vi "SwerveDrivePoseEst_New.vi"(4 "ModulePositions":T1[](array[typedef]) {"Angle"."SIN" format="%13.4f"; "Angle"."COS" format="%13.4f"; "Angle"."VALUE" format="%13.4f"}, 5 "gyroAngle":T2={"VALUE"=0.0, "COS"=1.0, "SIN"=0.0} {"SIN" format="%13.4f"; "COS" format="%13.4f"; "VALUE" format="%13.4f"}, 6 "SwerveKinematics":T3 {"SavedModuleStates"."Angle"."SIN" format="%13.4f"; "SavedModuleStates"."Angle"."COS" format="%13.4f"; "SavedModuleStates"."Angle"."VALUE" format="%13.4f"; "PrevCoR"."Y" format="%14.3f"; "PrevCoR"."X" format="%14.3f"; "Modules"."Y" format="%14.3f"; "Modules"."X" format="%14.3f"}, 7 "InitialPose":T7={"TRANSLATION"={"X"=0.0, "Y"=0.0}, "ROTATION"={"VALUE"=0.0, "COS"=1.0, "SIN"=0.0}} {"ROTATION"."SIN" format="%13.4f"; "ROTATION"."COS" format="%13.4f"; "ROTATION"."VALUE" format="%13.4f"; "TRANSLATION"."Y" format="%14.3f"; "TRANSLATION"."X" format="%14.3f"}, 8 "dt_Seconds":dbl=0.02, 9 "VisionMeasurementStdDevs":T4, 10 "LocalMeasurementStdDevs":T4, 11 "StateStdDevs":T4) -> (0 "Error":errorcluster, 3 "SwerveDrivePoseEstimate":T8={"M_VisionContR"=[], "m_nominal_dT"=0.0, "m_PrevTime_Sec"=0.0, "m_GyroOffset"={"VALUE"=0.0, "COS"=1.0, "SIN"=0.0}, "m_PrevAngle"={"VALUE"=0.0, "COS"=1.0, "SIN"=0.0}, "m_Observer"={"m_P"=[], "m_xHat"=[], "States"=0, "Outputs"=0, "m_ContR"=[], "m_ContQ"=[], "m_SigmasF"=[], "m_dT_Sec"=0.0, "MERWE_SCALED_SIGMA_PTS"={"m_Wm"=[], "States"=0, "Alpha"=0.0, "m_Wc"=[], "Kappa"=0}, "meanFuncX"=refnum, "meanFuncY"=refnum, "residualFuncX"=refnum, "residualFuncY"=refnum, "addFuncX"=refnum, "addFuncXExtra"=variant, "residualFuncYExtra"=variant, "residualFuncXExtra"=variant, "MeanFuncYExtra"=variant, "MeanFuncXExtra"=variant, "Inputs"=0}, "m_kinematics"={"NumModules"=0, "InverseKinematics"=[], "ForwardKinematics"=[], "Modules"=[], "PrevCoR"={"X"=0.0, "Y"=0.0}, "SavedModuleStates"=[]}, "Pose_Buffer"={"TimeStamps"=[], "Pose"=[], "Min_TimeStamp"=0.0, "Max_TimeStamp"=0.0, "ItemCount"=0, "MaxBufferTime"=0.0}, "States"=0, "Inputs"=0, "Outputs"=0} {"Pose_Buffer"."Pose"."ROTATION"."SIN" format="%13.4f"; "Pose_Buffer"."Pose"."ROTATION"."COS" format="%13.4f"; "Pose_Buffer"."Pose"."ROTATION"."VALUE" format="%13.4f"; "Pose_Buffer"."Pose"."TRANSLATION"."Y" format="%14.3f"; "Pose_Buffer"."Pose"."TRANSLATION"."X" format="%14.3f"; "m_kinematics"."SavedModuleStates"."Angle"."SIN" format="%13.4f"; "m_kinematics"."SavedModuleStates"."Angle"."COS" format="%13.4f"; "m_kinematics"."SavedModuleStates"."Angle"."VALUE" format="%13.4f"; "m_kinematics"."PrevCoR"."Y" format="%14.3f"; "m_kinematics"."PrevCoR"."X" format="%14.3f"; "m_kinematics"."Modules"."Y" format="%14.3f"; "m_kinematics"."Modules"."X" format="%14.3f"; "m_PrevAngle"."SIN" format="%13.4f"; "m_PrevAngle"."COS" format="%13.4f"; "m_PrevAngle"."VALUE" format="%13.4f"; "m_GyroOffset"."SIN" format="%13.4f"; "m_GyroOffset"."COS" format="%13.4f"; "m_GyroOffset"."VALUE" format="%13.4f"})   [LabVIEW 2019, in "Trajectory_Library.lvlib"]
doc: "Constructs a SwerveDrivePoseEstimator.\n\nThis class wraps an UnscentedKalmanFilter Unscented Kalman Filter to fuse latency-compensated vision measurements with swerve drive encoder velocity measurements. It will correct for noisy measurements and encoder drift. It is intended to be an easy but more accurate drop-in for SwerveDriveOdometry.\n \nSwerveDrivePoseEstimator_update should be called every robot loop. If your loops are faster or slower than the default of 0.02s, then you should change the nominal delta time using the calling parameter. \n \nSwerveDrivePoseEstimator_addVisionMeasurement can be called as infrequently as you want; if you never call it, then this class will behave mostly like regular encoder odometry.\n \nThe state-space system used internally has the following states (x), inputs (u), and outputs\n(y):\n \n x = [x, y, theta]? \n in the field coordinate system containing x position, \n y position, and heading.\n \n u = [v_l, v_r, dtheta]? \n containing left wheel velocity, right wheel velocity, \n and change in gyro heading.\n \n y = [x, y, theta]?\n from vision containing x position, y position, and\n heading; or <strong> y = [theta]? </strong> containing \n gyro heading.\n \n \nInputs:\n - gyroAngle -- The current gyro angle.\n - initialPoseMeters -- The starting pose estimate.\n - stateStdDevs -- Standard deviations of model states. Increase these numbers \n to trust your model's state estimates less. This matrix is in the form \n [x, y, theta]?, with units in meters and radians.\n - localMeasurementStdDevs -- Standard deviations of the encoder and gyro \n measurements. Increase these numbers to trust sensor readings from encoders \n and gyros less. This matrix is in the form [theta], with units in radians.\n - visionMeasurementStdDevs -- Standard deviations of the vision measurements. \n Increase these numbers to trust global measurements from vision less. \n This matrix is in the form [x, y,theta]?, with units in meters and radians.\n - nominalDtSeconds -- The time in seconds between each robot loop.\n - SwerveKinematics -- A correctly-configured kinematics object for your drivetrain.\n\n\nOutputs:\n - outSwevePoseEst -- Updated data cluster \n - Error -- If TRUE, an error occured."
uses:
  Trajectory_Library.lvlib
  TypeDef/SWERVE_DRIVE_POSE_EST.ctl
  <vilib>/Analysis/Matrix/Datatypes/RealMatrix.ctl
  TypeDef/ROTATION2D.ctl
  TypeDef/UNSCENTED_KALMAN_FILTER.ctl
  TypeDef/MERWE_SCALED_SIGMA_PTS.ctl
  TypeDef/CALLBACK_FUNC_TYPE.ctl
  TypeDef/SWERVE_DRIVE_KINEMATICS.ctl
  TypeDef/TRANSLATION2D.ctl
  TypeDef/SWERVE_DRIVE_MODULE_STATE.ctl
  TypeDef/TIME_INTERPOLATABLE_POSE2D.ctl
  TypeDef/POSE2D.ctl
  MatBuilder_Create.vi
  VecBuilder_3x1Fill.vi
  Pose2d_getXYAngle.vi
  Rotation2d_UnaryMinus.vi
  Rotation2d_RotateBy.vi
  Rotation2d_CreateAngle.vi
  Rotation2d_CreateXY.vi
  Util_CalcDist.vi
  <vilib>/Analysis/Matrix/NI_Matrix.lvlib
  TypeDef/SWERVE_DRIVE_MODULE_POSITION.ctl
panel:
  in  "RightDistance_M":dbl=0.02
  in  "LeftDistance_M":dbl=0.02
  # "<5,1>"
  # "<3, 1>"
  # "<3, 1>"
  # "<3, 3>"
  # "State Estimate <Statess,1>"
  # "<States, States>"
  # "<States, ?>"
  # "<Statess,  States>"
  # "<Outputs, Outputs>"
  # "<?, 1>"
  # "<?, 1>"
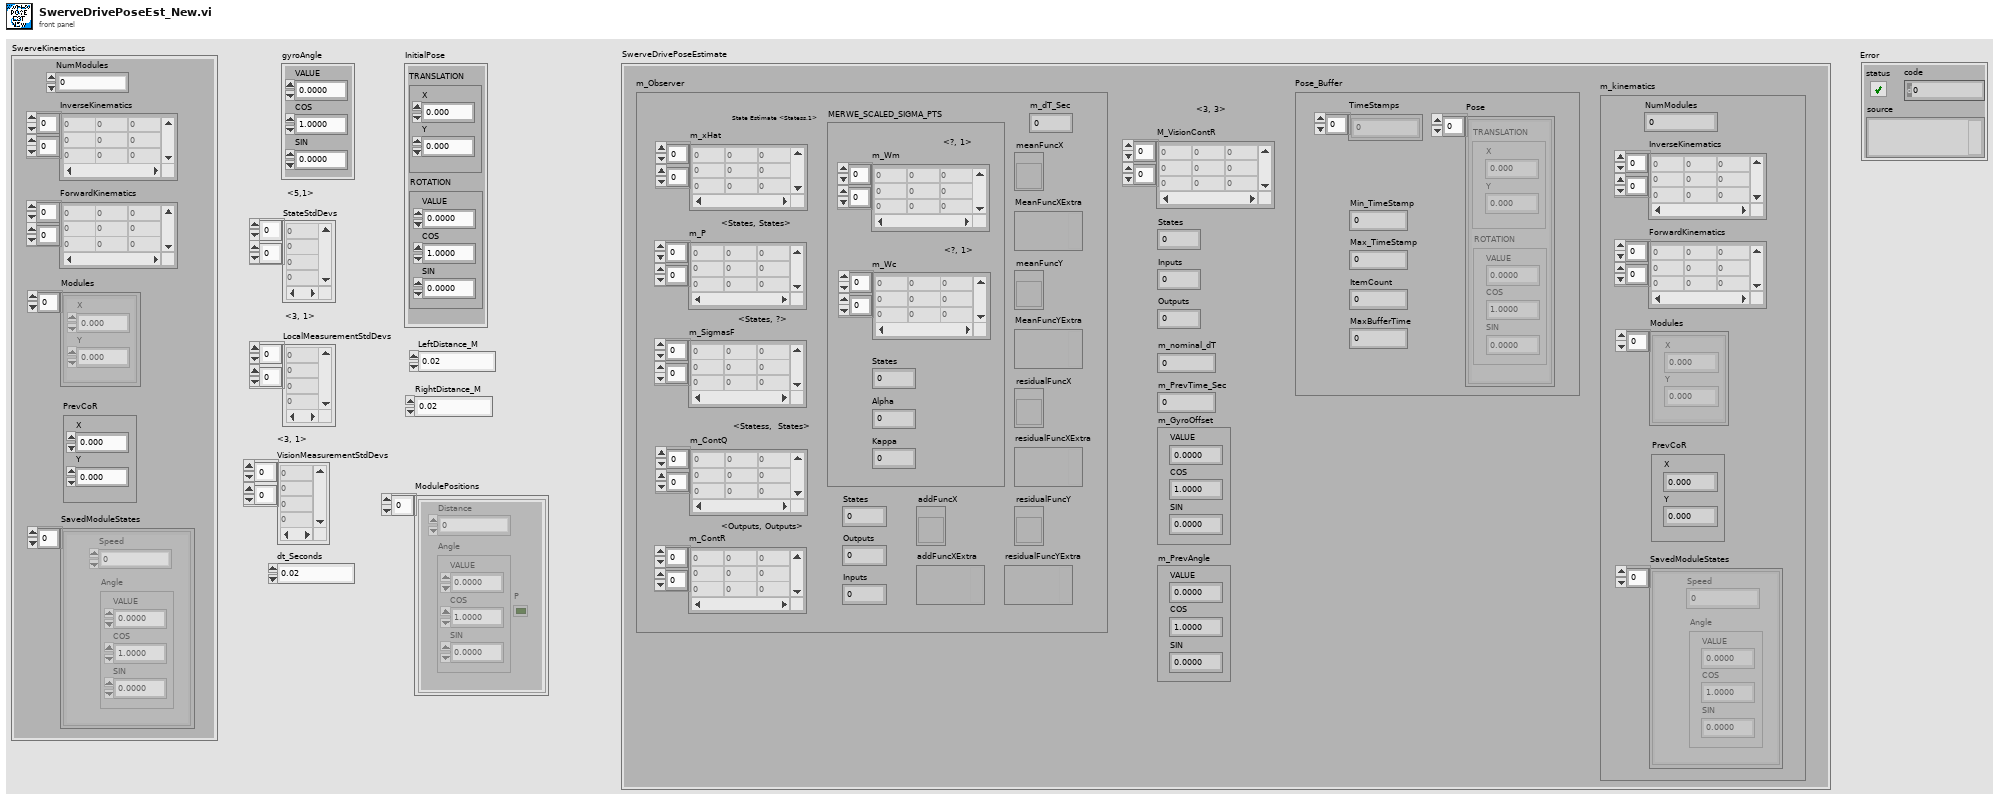
[diagram p1: front panel]
types:
  T1 = typedef "Trajectory_Library.lvlib/SWERVE_DRIVE_MODULE_POSITION.ctl" = cluster{"Distance":dbl, "Angle":T2, "P":bool}
  T2 = typedef "Trajectory_Library.lvlib/ROTATION2D.ctl" = cluster{"VALUE":dbl, "COS":dbl, "SIN":dbl}
  T3 = typedef "Trajectory_Library.lvlib/SWERVE_DRIVE_KINEMATICS.ctl" = cluster{"NumModules":i32, "InverseKinematics":T4, "ForwardKinematics":T4, "Modules":T5[], "PrevCoR":T5, "SavedModuleStates":T6[]}
  T4 = typedef "NI_Matrix.lvlib/RealMatrix.ctl" = dbl[][]
  T5 = typedef "Trajectory_Library.lvlib/TRANSLATION2D.ctl" = cluster{"X":dbl, "Y":dbl}
  T6 = typedef "Trajectory_Library.lvlib/SWERVE_DRIVE_MODULE_STATE.ctl" = cluster{"Speed":dbl, "Angle":T2}
  T7 = typedef "Trajectory_Library.lvlib/POSE2D.ctl" = cluster{"TRANSLATION":T5, "ROTATION":T2}
  T8 = typedef "Trajectory_Library.lvlib/SWERVE_DRIVE_POSE_EST.ctl" = cluster{"M_VisionContR":T4, "m_nominal_dT":dbl, "m_PrevTime_Sec":dbl, "m_GyroOffset":T2, "m_PrevAngle":T2, "m_Observer":T9, "m_kinematics":T3, "Pose_Buffer":T12, "States":i32, "Inputs":i32, "Outputs":i32}
  T9 = typedef "Trajectory_Library.lvlib/UNSCENTED_KALMAN_FILTER.ctl" = cluster{"m_P":T4, "m_xHat":T4, "States":i32, "Outputs":i32, "m_ContR":T4, "m_ContQ":T4, "m_SigmasF":T4, "m_dT_Sec":dbl, "MERWE_SCALED_SIGMA_PTS":T10, "meanFuncX":T11, "meanFuncY":T11, "residualFuncX":T11, "residualFuncY":T11, "addFuncX":T11, "addFuncXExtra":variant, "residualFuncYExtra":variant, "residualFuncXExtra":variant, "MeanFuncYExtra":variant, "MeanFuncXExtra":variant, "Inputs":i32}
  T10 = typedef "Trajectory_Library.lvlib/MERWE_SCALED_SIGMA_PTS.ctl" = cluster{"m_Wm":T4, "States":i32, "Alpha":dbl, "m_Wc":T4, "Kappa":i32}
  T11 = typedef "Trajectory_Library.lvlib/CALLBACK_FUNC_TYPE.ctl" = refnum<vi>
  T12 = typedef "Trajectory_Library.lvlib/TIME_INTERPOLATABLE_POSE2D.ctl" = cluster{"TimeStamps":dbl[], "Pose":T7[], "Min_TimeStamp":dbl, "Max_TimeStamp":dbl, "ItemCount":i32, "MaxBufferTime":dbl}
  T13 = typedef "Trajectory_Library.lvlib/UNSCENTED_KALMAN_NEW_FUNC_GROUP.ctl" = cluster{"meanFuncX":T11, "meanFuncY":T11, "residualFuncX":T11, "residualFuncY":T11, "addFuncX":T11, "MeanFuncXExtra":variant, "MeanFuncYExtra":variant, "residualFuncXExtra":variant, "residualFuncYExtra":variant, "addFuncXExtra":variant}
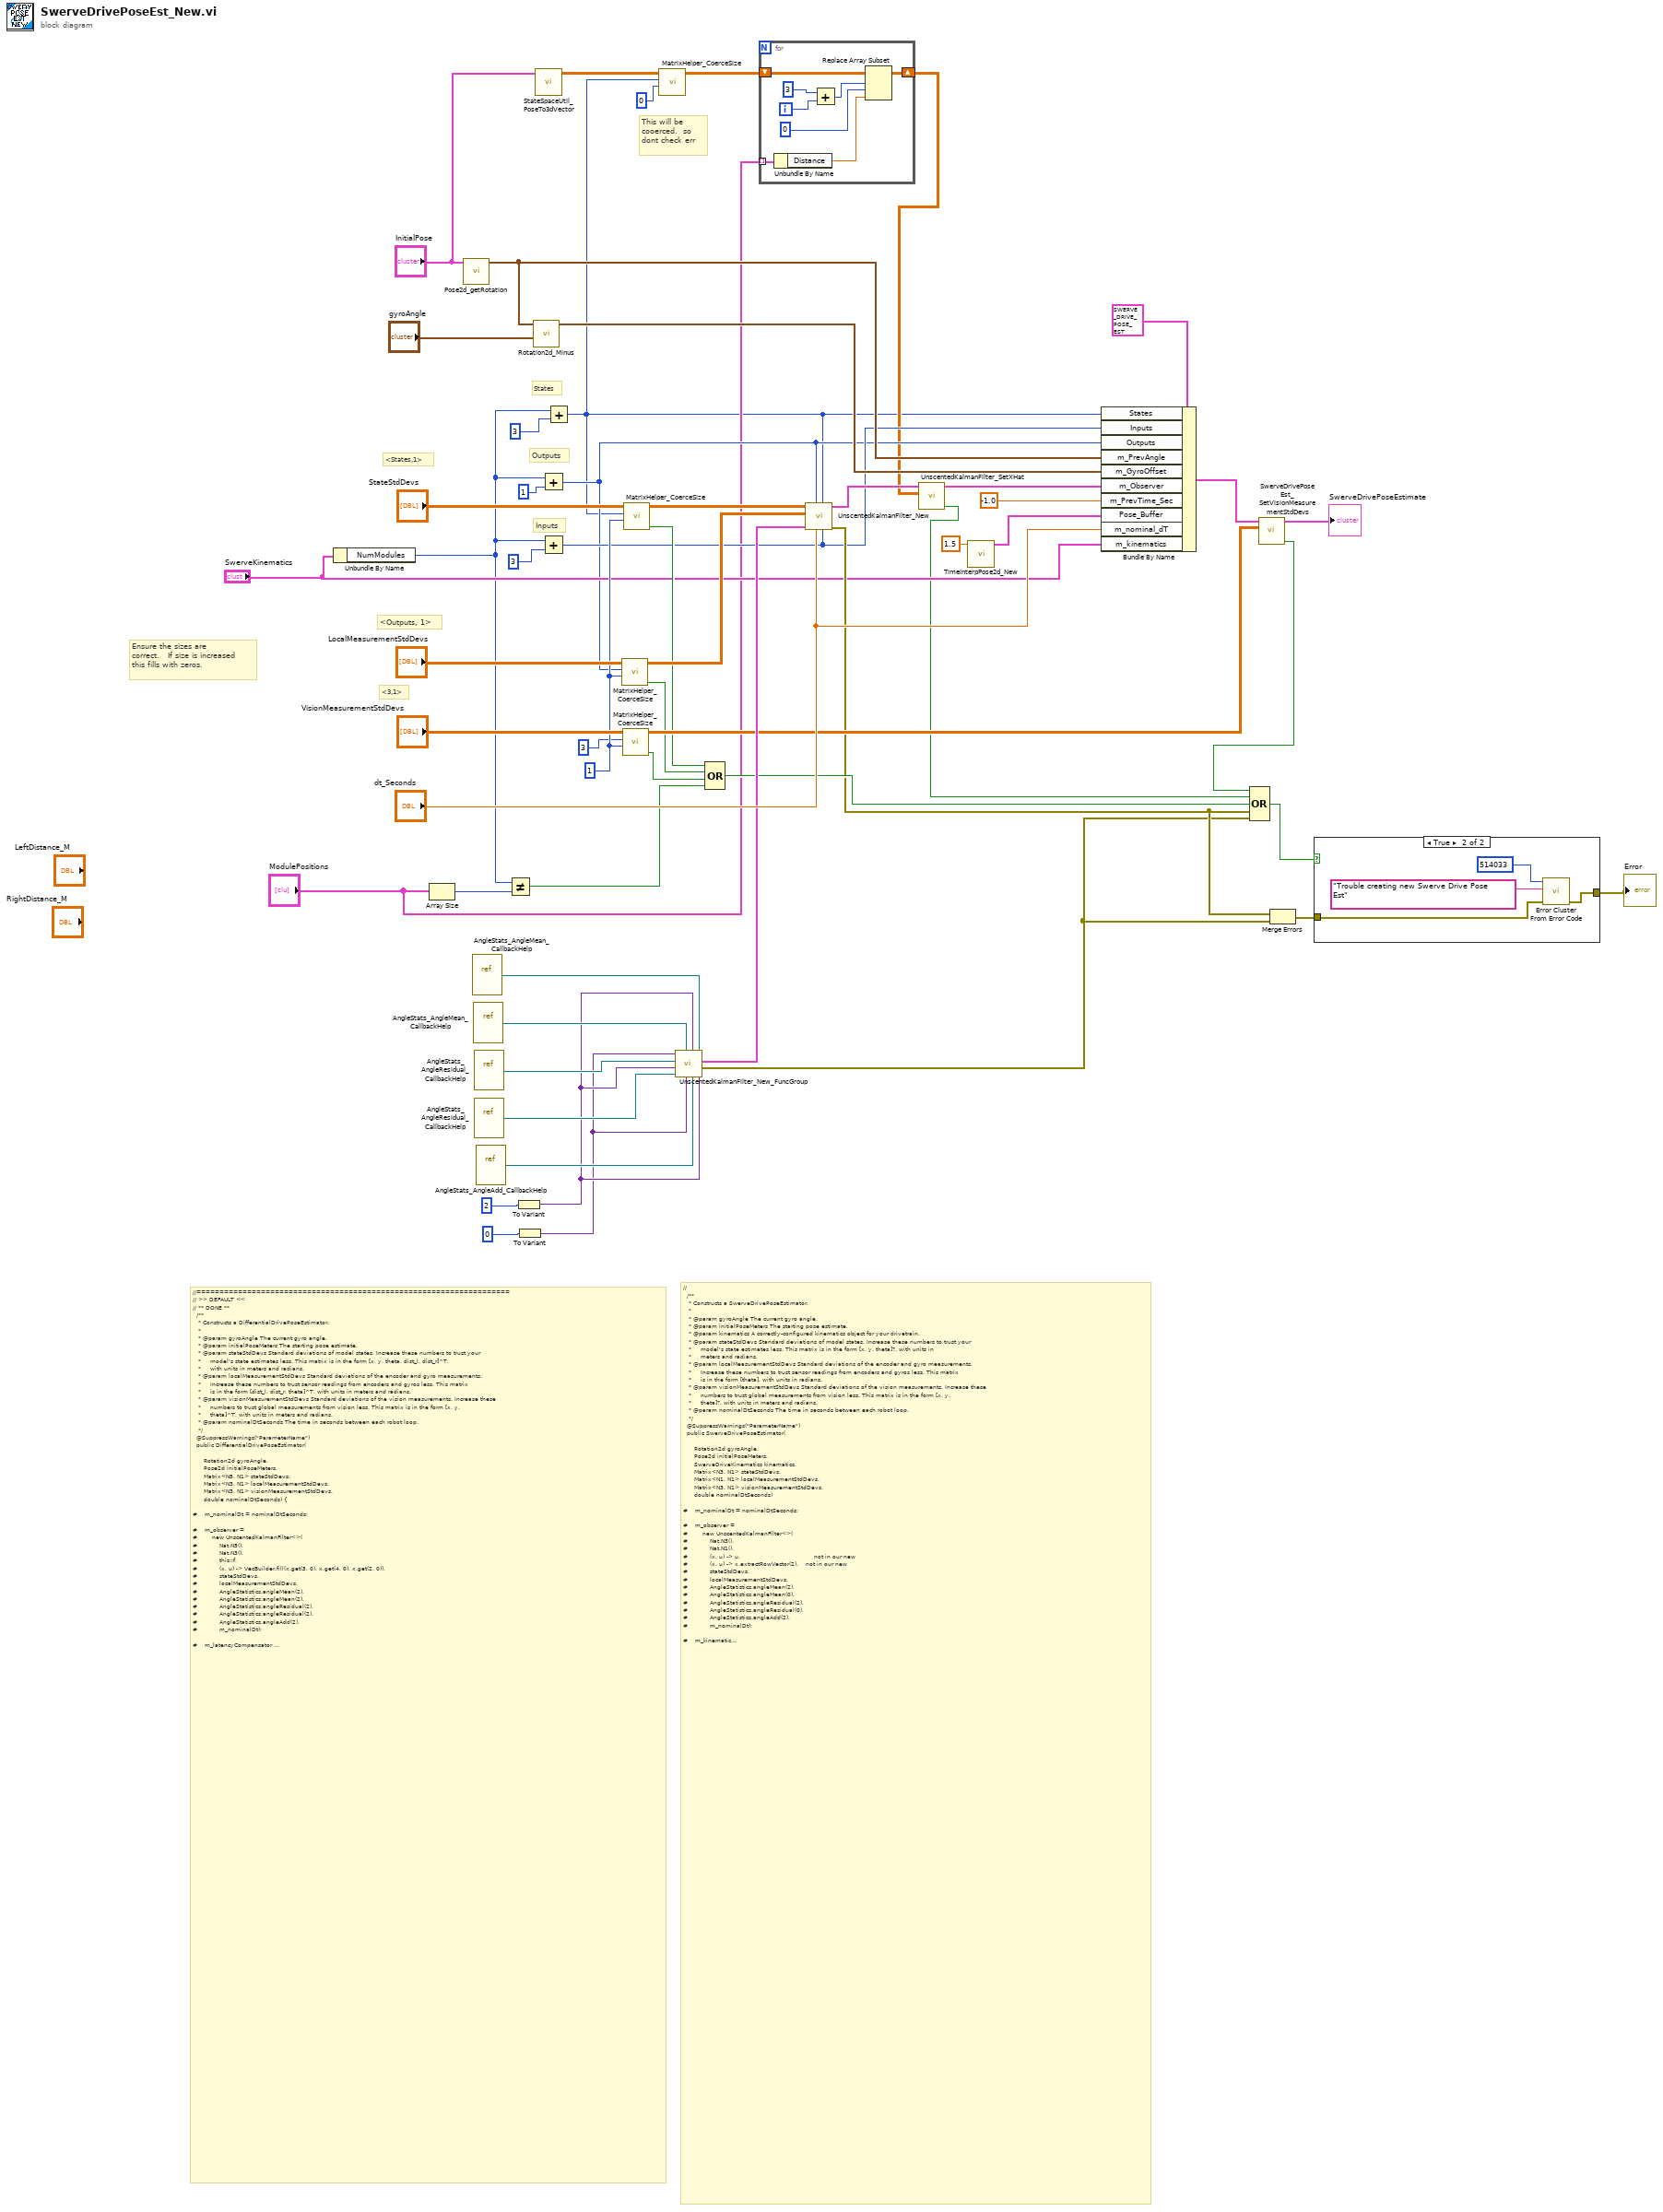
[diagram p0: block diagram]
diagram:
  w33 = 1 ("y")
  # "This will be\ncooerced.  so\ndont check err"
  # "<3,1>"
  # "//====================================================================\n// >> DEFAULT <<\n// ** DONE **\n  /**\n   * Constructs a DifferentialDrivePoseEstimator.\n   *\n   * @param gyroAngle The current gyro angle.\n   * @param initialPoseMeters The starting pose estimate.\n   * @param stateStdDevs Standard deviations of model states. Increase these numbers to trust your\n   *     model's state estimates less. This matrix is in the form [x, y, theta, dist_l, dist_r]^T,\n   *     with units in meters and radians.\n   * @param localMeasurementStdDevs Standard deviations of the encoder and gyro measurements.\n   *     Increase these numbers to trust sensor readings from encoders and gyros less. This matrix\n   *     is in the form [dist_l, dist_r, theta]^T, with units in meters and radians.\n   * @param visionMeasurementStdDevs Standard deviations of the vision measurements. Increase these\n   *     numbers to trust global measurements from vision less. This matrix is in the form [x, y,\n   *     theta]^T, with units in meters and radians.\n   * @param nominalDtSeconds The time in seconds between each robot loop.\n   */\n  @SuppressWarnings(\"ParameterName\")\n  public DifferentialDrivePoseEstimator(\n\n      Rotation2d gyroAngle,\n      Pose2d initialPoseMeters,\n      Matrix<N5, N1> stateStdDevs,\n      Matrix<N3, N1> localMeasurementStdDevs,\n      Matrix<N3, N1> visionMeasurementStdDevs,\n      double nominalDtSeconds) {\n\n#    m_nominalDt = nominalDtSeconds;\n\n#    m_observer =\n#        new UnscentedKalmanFilter<>(\n#            Nat.N5(),\n#            Nat.N3(),\n#            this::f,\n#            (x, u) -> VecBuilder.fill(x.get(3, 0), x.get(4, 0), x.get(2, 0)),\n#            stateStdDevs,\n#            localMeasurementStdDevs,\n#            AngleStatistics.angleMean(2),\n#            AngleStatistics.angleMean(2),\n#            AngleStatistics.angleResidual(2),\n#            AngleStatistics.angleResidual(2),\n#            AngleStatistics.angleAdd(2),\n#            m_nominalDt);\n\n#    m_latencyCompensator = new KalmanFilterLatencyCompensator<>();\n\n#    // Initialize vision R\n#    setVisionMeasurementStdDevs(visionMeasurementStdDevs);\n\n//JAS not part of the data structure....\n    m_visionCorrect =\n        (u, y) ->\n            m_observer.correct(\n                Nat.N3(),\n                u,\n                y,\n                (x, u1) -> new Matrix<>(x.getStorage().extractMatrix(0, 3, 0, 1)),\n                m_visionDiscreteR,\n                AngleStatistics.angleMean(2),\n                AngleStatistics.angleResidual(2),\n                AngleStatistics.angleResidual(2),\n                AngleStatistics.angleAdd(2));\n\n#    m_gyroOffset = initialPoseMeters.getRotation().minus(gyroAngle);\n#    m_previousAngle = initialPoseMeters.getRotation();\n#    m_observer.setXhat(fillStateVector(initialPoseMeters, 0.0, 0.0));\n  }"
  # "// \n  /**\n   * Constructs a SwerveDrivePoseEstimator.\n   *\n   * @param gyroAngle The current gyro angle.\n   * @param initialPoseMeters The starting pose estimate.\n   * @param kinematics A correctly-configured kinematics object for your drivetrain.\n   * @param stateStdDevs Standard deviations of model states. Increase these numbers to trust your\n   *     model's state estimates less. This matrix is in the form [x, y, theta]?, with units in\n   *     meters and radians.\n   * @param localMeasurementStdDevs Standard deviations of the encoder and gyro measurements.\n   *     Increase these numbers to trust sensor readings from encoders and gyros less. This matrix\n   *     is in the form [theta], with units in radians.\n   * @param visionMeasurementStdDevs Standard deviations of the vision measurements. Increase these\n   *     numbers to trust global measurements from vision less. This matrix is in the form [x, y,\n   *     theta]?, with units in meters and radians.\n   * @param nominalDtSeconds The time in seconds between each robot loop.\n   */\n  @SuppressWarnings(\"ParameterName\")\n  public SwerveDrivePoseEstimator(\n\n      Rotation2d gyroAngle,\n      Pose2d initialPoseMeters,\n      SwerveDriveKinematics kinematics,\n      Matrix<N3, N1> stateStdDevs,\n      Matrix<N1, N1> localMeasurementStdDevs,\n      Matrix<N3, N1> visionMeasurementStdDevs,\n      double nominalDtSeconds) \n\n#    m_nominalDt = nominalDtSeconds;\n\n#    m_observer =\n#        new UnscentedKalmanFilter<>(\n#            Nat.N3(),\n#            Nat.N1(),\n#            (x, u) -> u,                                        not in our new\n#            (x, u) -> x.extractRowVector(2),    not in our new\n#            stateStdDevs,\n#            localMeasurementStdDevs,\n#            AngleStatistics.angleMean(2),\n#            AngleStatistics.angleMean(0),\n#            AngleStatistics.angleResidual(2),\n#            AngleStatistics.angleResidual(0),\n#            AngleStatistics.angleAdd(2),\n#            m_nominalDt);\n\n#    m_kinematics = kinematics;\n\n#    m_latencyCompensator = new KalmanFilterLatencyCompensator<>();\n\n#    // Initialize vision R\n#    setVisionMeasurementStdDevs(visionMeasurementStdDevs);\n\n//JAS not part of the data structure....\n    m_visionCorrect =\n        (u, y) ->\n            m_observer.correct(\n                Nat.N3(),\n                u,\n                y,\n                (x, u1) -> x,\n                m_visionContR,\n                AngleStatistics.angleMean(2),\n                AngleStatistics.angleResidual(2),\n                AngleStatistics.angleResidual(2),\n                AngleStatistics.angleAdd(2));\n\n#    m_gyroOffset = initialPoseMeters.getRotation().minus(gyroAngle);\n#    m_previousAngle = initialPoseMeters.getRotation();\n#    m_observer.setXhat(  StateSpaceUtil.poseTo3dVector(initialPoseMeters));\n  }"
  # "Inputs"
  # "Outputs"
  # "States"
  # "<Outputs, 1>"
  # "<States,1>"
  # "Ensure the sizes are\ncorrect.   If size is increased \nthis fills with zeros."
  n1 = Unbundle By Name("SwerveKinematics") -> ("NumModules"=w14:i32)
  n2 = Array Size(array="ModulePositions") -> (size(s)=w13:i32)
  n3 = call "Pose2d_getRotation.vi"("in POSE"="InitialPose") -> ("out ROTATION"=w53:T2)  [unwired: 10 in]
  n4 = vi-ref "AngleStats_AngleMean_CallbackHelp.vi"() -> (w46:refnum<vi>)
  n5 = vi-ref "AngleStats_AngleMean_CallbackHelp.vi"() -> (w45:refnum<vi>)
  n6 = vi-ref "AngleStats_AngleResidual_CallbackHelp.vi"() -> (w44:refnum<vi>)
  n7 = vi-ref "AngleStats_AngleResidual_CallbackHelp.vi"() -> (w43:refnum<vi>)
  n8 = vi-ref "AngleStats_AngleAdd_CallbackHelp.vi"() -> (w41:refnum<vi>)
  n9 = Not Equal?(x=w14, y=w13) -> (x != y?=w12:bool)
  n10 = To Variant(anything=2) -> (Variant=w40:variant)
  n11 = To Variant(anything=0) -> (Variant=w27:variant)
  n12 = call "Rotation2d_Minus.vi"("other ROTATION"="gyroAngle", "in ROTATION"=w53) -> ("out ROTATION"=w54:T2)  [unwired: 9 in]
  n13 = call "StateSpaceUtil_PoseTo3dVector.vi"("Pose"="InitialPose") -> ("Pose Vector"=w4:T4)  [unwired: 10 in]
  n14 = Add(x=w14, y=1 ("Outputs")) -> (x+y=w10:i32)
  n15 = Add(x=w14, y=3 ("Inputs")) -> (x+y=w11:i32)
  n16 = Add(x=w14, y=3 ("States")) -> (x+y=w1:i32)
  n17 = call "MatrixHelper_CoerceSize.vi"("Columns"=w33, "Rows"=w10, "input matrix"="LocalMeasurementStdDevs") -> ("Coerced"=w30:bool, "output matrix"=w38:T4)  [unwired: 7 in]
  n18 = call "MatrixHelper_CoerceSize.vi"("Columns"=w33, "Rows"=3, "input matrix"="VisionMeasurementStdDevs") -> ("Coerced"=w29:bool, "output matrix"=w34:T4)  [unwired: 7 in]
  n19 = call "MatrixHelper_CoerceSize.vi"("Columns"=w33, "Rows"=w1, "input matrix"="StateStdDevs") -> ("Coerced"=w31:bool, "output matrix"=w36:T4)  [unwired: 7 in]
  n20 = call "MatrixHelper_CoerceSize.vi"("Columns"=0, "Rows"=w1, "input matrix"=w4) -> ("output matrix"=w3:T4)  [unwired: 7 in, 1 out]
  n21 = call "UnscentedKalmanFilter_New_FuncGroup.vi"("addFuncXExtra"=w40, "MeanFuncX"=w46, "AddFuncX"=w41, "MeanFuncXExtra"=w40, "residualFuncYExtra"=w27, "MeanFuncY"=w45, "ResidualFuncY"=w43, "residualFuncXExtra"=w40, "ResidualFuncX"=w44, "MeanFuncYExtra"=w27) -> ("Error"=w22:errorcluster, "UNSCENTED_KALMAN_NEW_FUNC_GROUP"=w47:T13)
  n22 = Compound Arithmetic op=OR(w31, w30, w29, w12) -> (w32:bool)
  n23 = for {
    tunnel: "ModulePositions" -> [w65] mode=indexing
    shift-right: [w58] -> w7
    shift-left: w3 -> [w62]
    i -> [w63]
    n24 = Unbundle By Name(w65) -> ("Distance"=w59:dbl)
    n25 = Add(x=3 ("States"), y=w63) -> (x+y=w61:i32)
    n26 = Replace Array Subset(array=w62, new element=w59, index (row)=w61, index (col)=0 ("disabled index (col)")) -> (w58:T4)
  }
  n27 = call "UnscentedKalmanFilter_New.vi"("Inputs"=w11, "States"=w1, "dt_Seconds"="dt_Seconds", "Outputs"=w10, "UNSCENTED_KALMAN_NEW_FUNC_GROUP"=w47, "MeasurementStdDevs"=w38, "StateStdDevs"=w36) -> ("Error"=w23:errorcluster, "UnscentedKalmanFiilter"=w51:T9)  [unwired: 3 in]
  n28 = call "UnscentedKalmanFilter_SetXHat.vi"("xHat"=w7, "in UnscentedKalmanFiilter"=w51) -> ("SizeCoerced"=w6:bool, "out UnscentedKalmanFiilter"=w52:T9)  [unwired: 8 in]
  n29 = call "TimeInterpPose2d_New.vi"("MaxTime"=1.5) -> ("TimeInterpPose"=w19:T12)  [unwired: 10 in]
  n30 = Bundle By Name(cluster=T8 {"M_VisionContR"=[], "m_nominal_dT"=0.0, "m_PrevTime_Sec"=0.0, "m_GyroOffset"={"VALUE"=0.0, "COS"=1.0, "SIN"=0.0}, "m_PrevAngle"={"VALUE"=0.0, "COS"=1.0, "SIN"=0.0}, "m_Observer"={"m_P"=[], "m_xHat"=[], "States"=0, "Outputs"=0, "m_ContR"=[], "m_ContQ"=[], "m_SigmasF"=[], "m_dT_Sec"=0.0, "MERWE_SCALED_SIGMA_PTS"={"m_Wm"=[], "States"=0, "Alpha"=0.0, "m_Wc"=[], "Kappa"=0}, "meanFuncX"=refnum, "meanFuncY"=refnum, "residualFuncX"=refnum, "residualFuncY"=refnum, "addFuncX"=refnum, "addFuncXExtra"=variant, "residualFuncYExtra"=variant, "residualFuncXExtra"=variant, "MeanFuncYExtra"=variant, "MeanFuncXExtra"=variant, "Inputs"=0}, "m_kinematics"={"NumModules"=0, "InverseKinematics"=[], "ForwardKinematics"=[], "Modules"=[], "PrevCoR"={"X"=0.0, "Y"=0.0}, "SavedModuleStates"=[]}, "Pose_Buffer"={"TimeStamps"=[], "Pose"=[], "Min_TimeStamp"=0.0, "Max_TimeStamp"=0.0, "ItemCount"=0, "MaxBufferTime"=0.0}, "States"=0, "Inputs"=0, "Outputs"=0} ("DIFF_DRIVE_POSE_EST"), "States"=w1, "Inputs"=w11, "Outputs"=w10, "m_PrevAngle"=w53, "m_GyroOffset"=w54, "m_Observer"=w52, "m_PrevTime_Sec"=-1.0, "Pose_Buffer"=w19, "m_nominal_dT"="dt_Seconds", "m_kinematics"="SwerveKinematics") -> (w50:T8)
  n31 = call "SwerveDrivePoseEst_SetVisionMeasurementStdDevs.vi"("VisionMeasurementStdDevs"=w34, "in SwerveDrivePoseEstimate"=w50) -> ("Size Coerced"=w5:bool, "Out SwerveDrivePoseEstimate"=→"SwerveDrivePoseEstimate":T8)  [unwired: 8 in]
  n32 = Compound Arithmetic op=OR(w5, w6, w32, w23, w22) -> (w24:bool)
  n33 = Merge Errors(w23, w22) -> (w25:errorcluster)
  n34 = case shown="True" w24 {
    tunnel: w25 -> [w66 w69]
    tunnel: [w66 w70] -> w21
    frame False {
    }
    frame True {
      n35 = call <vilib>:"Error Cluster From Error Code.vi"("error in (no error)"=w69, "error message (\"\")"="Trouble creating new Swerve Drive Pose Est" ("error message (\"\")"), "error code (0)"=514033) -> ("error out"=w70:errorcluster)  [unwired: 6 in]
    }
  }
  "Error" <- w21
